vi "Get Source Node of Terminal.vi"(8 "error in (no error)":errorcluster, 11 "Terminal in":refnum<vi>) -> (0 "error out":errorcluster, 3 "Generic out":refnum<vi>)   [LabVIEW 2018, in "RPN.lvlib"]
uses:
  RPN.lvlib
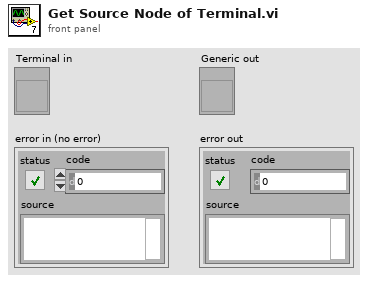
[diagram p1: front panel]
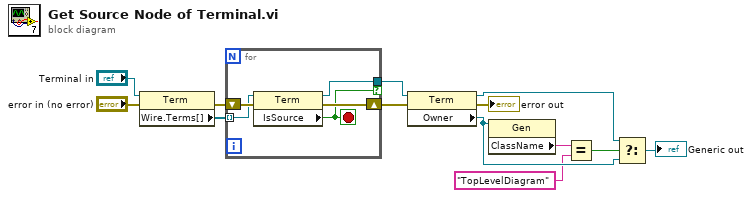
[diagram p0: block diagram]
diagram:
  n1 = property class="Term"(reference="Terminal in", error in="error in (no error)") -> (error out=w10:errorcluster, "Wire.Terms[]"=w8:refnum<vi>[])  [unwired: 1 out]
  n2 = for {
    tunnel: w8 -> [w16] mode=indexing
    tunnel: [w14] -> w11 if=w15
    shift-right: [w17] -> w12
    shift-left: w10 -> [w18]
    stop <- w15 stop-if-true
    n3 = property class="Term"(reference=w16, error in=w18) -> (reference out=w14:refnum<vi>, error out=w17:errorcluster, "IsSource"=w15:bool)
  }
  n4 = property class="Term"(reference=w11, error in=w12) -> (reference out=w4:refnum<vi>, error out=→"error out":errorcluster, "Owner"=w5:refnum<vi>)
  n5 = property class="Gen"(reference=w5) -> ("ClassName"=w2:string)  [unwired: 1 in, 2 out]
  n6 = Equal?(x=w2, y="TopLevelDiagram") -> (x = y?=w1:bool)
  n7 = Select(t=w4, s=w1, f=w5) -> (s? t:f=→"Generic out":refnum<vi>)
